vi "Pt Dist.vi"(10 "point b":cluster{"x":sgl, "y":sgl}, 11 "point a":cluster{"x":sgl, "y":sgl}) -> (3 "dist":sgl)   [LabVIEW 2020]
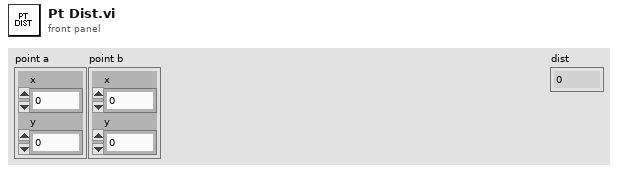
[diagram p1: front panel]
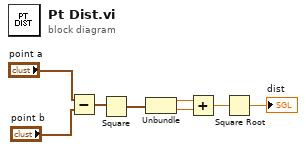
[diagram p0: block diagram]
diagram:
  n1 = Subtract(x="point a", y="point b") -> (x-y=w6:cluster{"x":sgl, "y":sgl})
  n2 = Square(x=w6) -> (x^2=w5:cluster{"x":sgl, "y":sgl})
  n3 = Unbundle(w5) -> ("x"=w4:sgl, "y"=w3:sgl)
  n4 = Add(x=w4, y=w3) -> (x+y=w2:sgl)
  n5 = Square Root(x=w2) -> (sqrt(x)=→"dist":sgl)
